vi "Destroy.vi"(8 "error in (no error)":errorcluster, 11 "User Interface in":refnum<class "User Interface.lvclass">) -> (0 "error out":errorcluster, 3 "User Interface out":refnum<class "User Interface.lvclass">)   [LabVIEW 2021, in "DSF Core.lvlib" / "User Interface.lvclass"]
uses:
  User Interface.lvclass
  User Interface.lvclass/User Interface.ctl
  Configuration/Configuration.lvclass
  User Interface Events/User Interface Events.lvclass
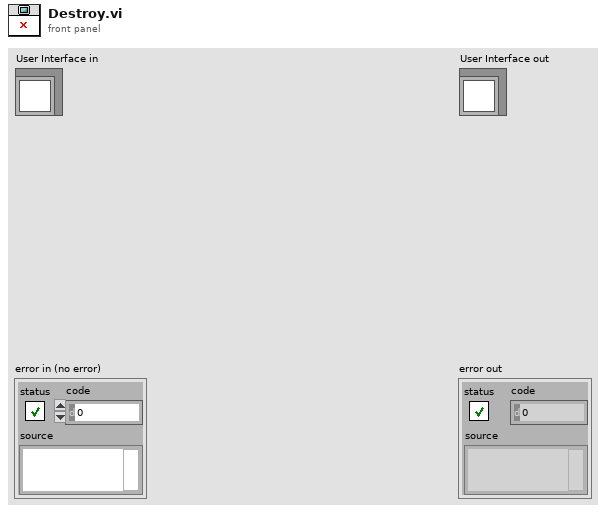
[diagram p1: front panel]
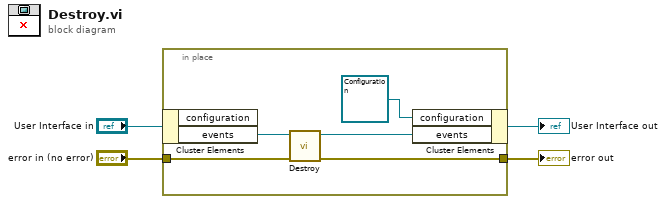
[diagram p0: block diagram]
diagram:
  n1 = in-place {
    in-place-border: "error in (no error)" -> [w6]
    in-place-border: [w5] -> w2
    n2 = in-place-cluster #1("User Interface in") -> ("events"=w9:refnum<class "User Interface Events.lvclass">)  [unwired: 1 out]
    n3 = call "Destroy.vi"("error in (no error)"=w6, "User Interface Events in"=w9) -> ("error out"=w5:errorcluster, "User Interface Events out"=w8:refnum<class "User Interface Events.lvclass">)  [unwired: 8 in]
    n4 = in-place-cluster #1("configuration"=refnum<class "Configuration.lvclass"> refnum, "events"=w8) -> (→"User Interface out":refnum<class "User Interface.lvclass">)
  }
  "error out" <- w2
